vi "event_start_stop.vi"(6 "Wavelet Array Length":i32, 10 "Event Indices":i32[](array[numeric])) -> (1 "Event End Time":dbl[](array[numeric]), 2 "Event Start Time":dbl[](array[numeric]))   [LabVIEW 2014]
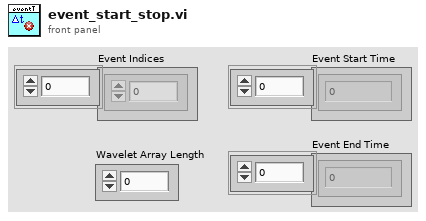
[diagram p1: front panel]
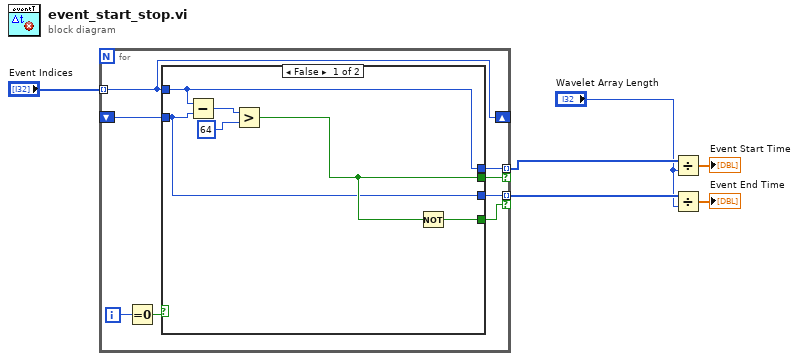
[diagram p0: block diagram]
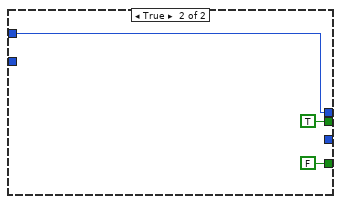
[diagram p2: hidden frame]
diagram:
  n1 = for {
    tunnel: "Event Indices" -> [w12] mode=indexing
    shift-right: [w12] -> _
    shift-left: _ -> [w13]
    tunnel: [w8] -> w5 mode=indexing if=w10
    tunnel: [w7] -> w3 mode=indexing if=w9
    i -> [w11]
    n2 = Equal To 0?(x=w11) -> (x = 0?=w14:bool)
    n3 = case shown="False" w14 {
      tunnel: w13 -> [w15 _]
      tunnel: w12 -> [w16 w21]
      tunnel: [w18 TRUE] -> w10
      tunnel: [w17 FALSE] -> w9
      tunnel: [w16 w21] -> w8
      tunnel: [w15 _] -> w7
      frame False {
        n4 = Subtract(x=w16, y=w15) -> (x-y=w20:i32)
        n5 = Greater?(x=w20, y=64) -> (0:w18:bool)
        n6 = Not(x=w18) -> (.not. x?=w17:bool)
      }
      frame True {
      }
    }
  }
  n7 = Divide(x=w5, y="Wavelet Array Length") -> (x/y=→"Event Start Time":dbl[])
  n8 = Divide(x=w3, y="Wavelet Array Length") -> (x/y=→"Event End Time":dbl[])
